vi "Prax8.vi"() -> ()   [LabVIEW 2020]
panel:
  out "Array":dbl[](array[numeric])
  in  "b 2":dbl=1000.0
  in  "module path 3":path=path "C:/ylesanne1.py"
  in  "sone sisend":string="tere"
  out "return value 2":string
  in  "module path 2":path=path "C:/ylesanne1.py"
  out "return value":dbl
  out "a väljund":i32
  out "b väjund":i32
  in  "b":i32=10
  in  "a":i32=10
  in  "module path":path=path "C:/ylesanne1.py"
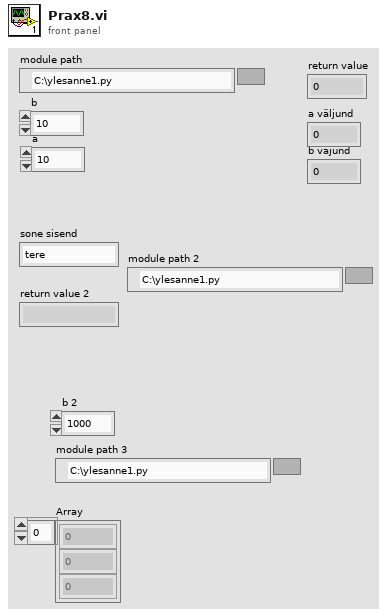
[diagram p1: front panel]
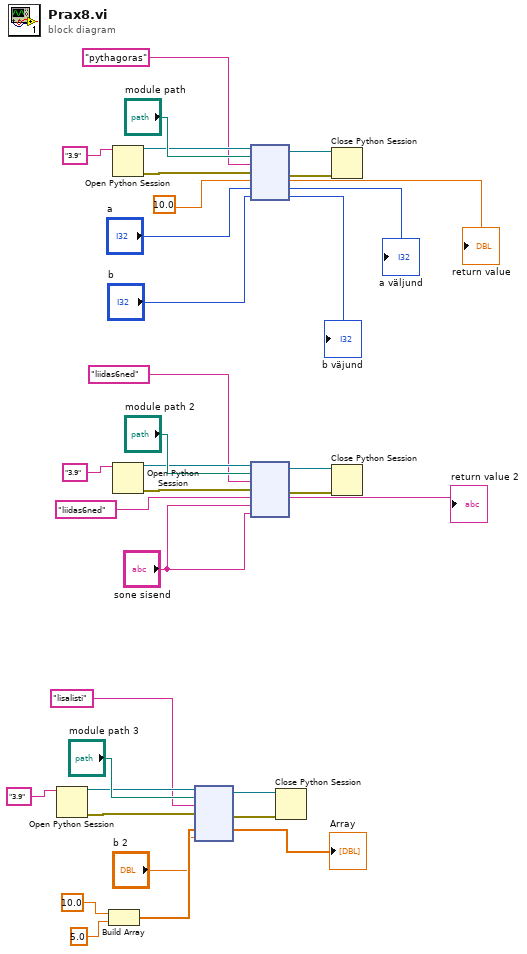
[diagram p0: block diagram]
diagram:
  n1 = Open Python Session(python version="3.9" ("Python version")) -> (session out=w10:refnum<k35>, error out=w9:errorcluster)  [unwired: 2 in]
  n2 = Build Array(10.0 ("element"), 5.0 ("element")) -> (w3:dbl[])
  n3 = Open Python Session(python version="3.9" ("Python version")) -> (session out=w33:refnum<k35>, error out=w32:errorcluster)  [unwired: 2 in]
  n4 = Open Python Session(python version="3.9" ("Python version")) -> (session out=w20:refnum<k35>, error out=w19:errorcluster)  [unwired: 2 in]
  n5 = node(w10, "module path 3", "lisalisti" ("function name"), w9, w3, "b 2") -> (w8:refnum<k35>, w7:errorcluster, →"Array":dbl[])  [unwired: 3 in, 2 out]
  n6 = node(w33, "module path", "pythagoras" ("function name"), w32, 10.0 ("a 2"), "a", "b") -> (w31:refnum<k35>, w30:errorcluster, →"return value":dbl, →"a väljund":i32, →"b väjund":i32)  [unwired: 2 out]
  n7 = node(w20, "module path 2", "liidas6ned" ("function name"), w19, "liidas6ned" ("function name"), "sone sisend", "sone sisend") -> (w18:refnum<k35>, w17:errorcluster, →"return value 2":string)  [unwired: 2 in, 2 out]
  n8 = Close Python Session(session in=w8, error in=w7) -> ()  [unwired: 1 out]
  n9 = Close Python Session(session in=w31, error in=w30) -> ()  [unwired: 1 out]
  n10 = Close Python Session(session in=w18, error in=w17) -> ()  [unwired: 1 out]
